vi "ABR3-Restore Defaults.vi"(7 "User":string) -> (4 "Params":T2={"CAP or ABR"=enum."ABR", "Stimulus"={"Ear"=enum."Left", "Waveform"=enum."TONE PIP", "Frequency (kHz)"="4", "Rep rate (/sec)"=30.0, "Alternate Polarity"=TRUE, "WavFiles"="", "Level (dB SPL)"=30.0, "WavFolder"=path "", "Chirp"={"Type"=enum."AN latency-corrected", "Duration (ms)"=0.0, "Fmin (kHz)"=0.0, "Fmax (kHz)"=0.0, "precompensate"=FALSE}, "Noise"={"Seed"=0, "InvFilt"=FALSE, "AWeight"=FALSE, "afile"=path "", "Filter"={"Type"=enum."Lowpass", "CF (kHz)"=0.0, "BW (kHz)"=0.0, "Cascade"=FALSE, "Quadrature"=FALSE, "Scale Factor"=0.0, "Stages"=[], "Class"=enum."Elliptic", "Order"=0, "BWUnits"=enum."Linear"}}}, "Masker"={"Filter"={"Type"=enum."Lowpass", "CF (kHz)"=0.0, "BW (kHz)"=0.0, "Cascade"=FALSE, "Quadrature"=FALSE, "Scale Factor"=0.0, "Stages"=[], "Class"=enum."Elliptic", "Order"=0, "BWUnits"=enum."Linear"}, "Use masker"=FALSE, "Level"={"Level"=0.0, "Units"=enum."dB atten", "Max"=0.0, "Multiplier"=0.0, "Cal File"=path "", "Cal"={"Freq (Hz)"=[], "Mag (dB SPL)"=[], "Phase (deg)"=[]}}, "Audiogram Comp"=FALSE, "Audiogram File"=path "", "InvFilt"=FALSE}, "Sequence"={"Start (dB)"=20, "Stop (dB)"=80, "Step (dB)"=5, "Var"=enum."Signal", "Order"=enum."Sequential"}, "Controls"={"on"=FALSE, "value"=0.0, "spacing"=0}, "Response"={"Gain"=10000, "Averages"=512, "Window (ms)"=8.5, "Thr Fast Steps"=1.5, "AI Fs"=25000.0}, "Hidden"={"AO Samp Rate Hz"=100000.0, "Duration (ms)"=5.0, "Ramp (ms)"=0.5, "Click width (us)"=100.0}} {"Response"."Thr Fast Steps" format="%.2f"; "Response"."Window (ms)" format="%.2f"; "Sequence"."Start (dB)" step=5}, 6 "Threshold Estimation":T1, 8 "settings":path=path "C:/Users/engr/Documents/EPL/CFTS/ABR/test.ini")   [LabVIEW 2020]
uses:
  TypeDefs/ABR3-Parameters.ctl
  TypeDefs/ABR3-Stimulus.ctl
  epl-vi-lib/Utility VIs/Type Defs/Left-Right ring.ctl
  TypeDefs/ABR-Waveform Enum.ctl
  epl-vi-lib/Signal Synthesis VIs/Controls/Advanced Filter XCtl/Advanced Filter XCtl.xctl
  TypeDefs/ABR3-Masker Spec.ctl
  epl-vi-lib/Signal Synthesis VIs/Controls/Level XCtl/Level XCtl.xctl
  TypeDefs/ABR3-Sequence Spec.ctl
  TypeDefs/ABR3-Controls.ctl
  TypeDefs/ABR3-Response.ctl
  TypeDefs/ABR3-Hidden Params.ctl
  Threshold Estimation VIs/ABR3-Threshold Estimation Parameters.ctl
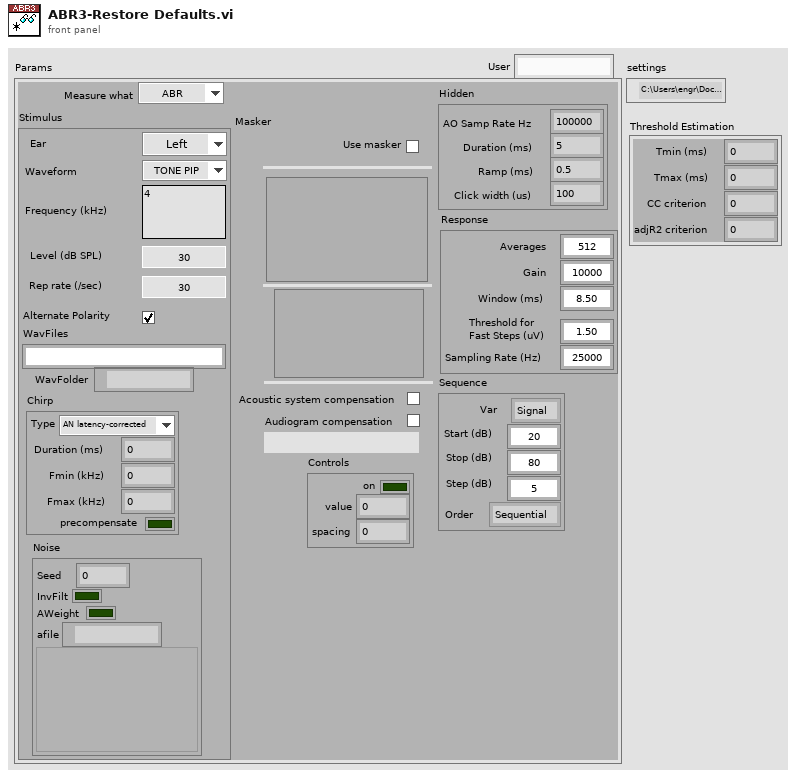
[diagram p1: front panel]
types:
  T1 = typedef "ABR3-Threshold Estimation Parameters.ctl" = cluster{"Tmin (ms)":dbl, "Tmax (ms)":dbl, "CC criterion":dbl, "adjR2 criterion":dbl}
  T2 = typedef "ABR3-Parameters.ctl" = cluster{"CAP or ABR":enum16{"CAP", "ABR"}, "Stimulus":T3, "Masker":T7, "Sequence":T9, "Controls":T10, "Response":T11, "Hidden":T12}
  T3 = typedef "ABR3-Stimulus.ctl" = cluster{"Ear":T4, "Waveform":T5, "Frequency (kHz)":string, "Rep rate (/sec)":dbl, "Alternate Polarity":bool, "WavFiles":string, "Level (dB SPL)":dbl, "WavFolder":path, "Chirp":cluster{"Type":enum16{"AN latency-corrected", "Arbitrary"}, "Duration (ms)":dbl, "Fmin (kHz)":dbl, "Fmax (kHz)":dbl, "precompensate":bool}, "Noise":cluster{"Seed":i32, "InvFilt":bool, "AWeight":bool, "afile":path, "Filter":cluster{"Type":enum16{"Lowpass", "Highpass", "Bandpass", "Bandstop", "OFF"}, "CF (kHz)":dbl, "BW (kHz)":dbl, "Cascade":bool, "Quadrature":bool, "Scale Factor":dbl, "Stages":cluster{"IIR Filter":cluster{"filter structure":enum32{"IIR 2nd Order", "IIR 4th Order"}, "Reverse Coefficients":dbl[], "Forward Coefficients":dbl[]}, "State":dbl[]}[], "Class":enum16{"Elliptic", "Butterworth"}, "Order":i32, "BWUnits":T6}}}
  T4 = typedef "Left-Right ring.ctl" = enum16{"Right", "Left"}
  T5 = typedef "ABR-Waveform Enum.ctl" = enum16{"TONE PIP", "CLICK", "FILE", "CHIRP", "NOISE", "VERHULST"}
  T6 = typedef "Filter-Bandwidth Units.ctl" = enum16{"Linear", "Octaves", "Min-Max"}
  T7 = typedef "ABR3-Masker Spec.ctl" = cluster{"Filter":cluster{"Type":enum16{"Lowpass", "Highpass", "Bandpass", "Bandstop", "OFF"}, "CF (kHz)":dbl, "BW (kHz)":dbl, "Cascade":bool, "Quadrature":bool, "Scale Factor":dbl, "Stages":cluster{"IIR Filter":cluster{"filter structure":enum32{"IIR 2nd Order", "IIR 4th Order"}, "Reverse Coefficients":dbl[], "Forward Coefficients":dbl[]}, "State":dbl[]}[], "Class":enum16{"Elliptic", "Butterworth"}, "Order":i32, "BWUnits":T6}, "Use masker":bool, "Level":cluster{"Level":dbl, "Units":T8, "Max":dbl, "Multiplier":dbl, "Cal File":path, "Cal":cluster{"Freq (Hz)":dbl[], "Mag (dB SPL)":dbl[], "Phase (deg)":dbl[]}}, "Audiogram Comp":bool, "Audiogram File":path, "InvFilt":bool}
  T8 = typedef "Level Units.ctl" = enum16{"dB atten", "dB SPL", "dB re 1 Vrms", "dB V/Hz½", "mW", "dB HL", "Volts", "dB mW"}
  T9 = typedef "ABR3-Sequence Spec.ctl" = cluster{"Start (dB)":i32, "Stop (dB)":i32, "Step (dB)":i32, "Var":enum16{"Signal", "Masker"}, "Order":enum16{"Sequential", "Random"}}
  T10 = typedef "ABR3-Controls.ctl" = cluster{"on":bool, "value":dbl, "spacing":i32}
  T11 = typedef "ABR3-Response.ctl" = cluster{"Gain":i32, "Averages":i32, "Window (ms)":sgl, "Thr Fast Steps":sgl, "AI Fs":dbl}
  T12 = typedef "ABR3-Hidden Params.ctl" = cluster{"AO Samp Rate Hz":dbl, "Duration (ms)":dbl, "Ramp (ms)":dbl, "Click width (us)":dbl}
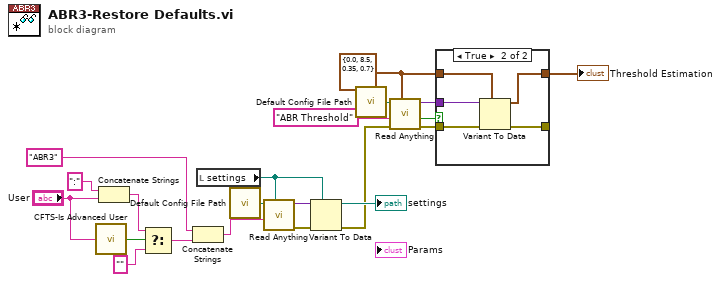
[diagram p0: block diagram]
diagram:
  w3 = T1 {"Tmin (ms)"=0.0, "Tmax (ms)"=8.5, "CC criterion"=0.35, "adjR2 criterion"=0.7} ("Threshold Estimation")
  n1 = call "CFTS-Is Advanced User.vi"("Experimenter"="User") -> ("Advanced user"=w17:bool)
  n2 = Concatenate Strings(":" ("string"), "User") -> (w14:string)
  n3 = Select(t=w14, s=w17, f="") -> (s? t:f=w12:string)
  n4 = Concatenate Strings("ABR3" ("Section Name (Name of \"Type of Anything\")"), w12) -> (w10:string)
  n5 = local read "settings"() -> (w19:path)
  n6 = call "Default Config File Path.vi"() -> ("Default config file name"=w20:path)
  n7 = call "Read Anything.vi"("Type of Anything"=w19, "Section Name (Name of \"Type of Anything\")"=w10, "Path (dialog)"=w20) -> ("Error Out"=w9:errorcluster, "Anything"=w21:variant)  [unwired: 6 in, 1 out]
  n8 = Variant To Data(error in=w9, type=w19, Variant=w21) -> (data=→"settings":path, error out=w2:errorcluster)
  n9 = call "Default Config File Path.vi"() -> ("Default config file name"=w8:path)
  n10 = call "Read Anything.vi"("Type of Anything"=w3, "Error In"=w2, "Section Name (Name of \"Type of Anything\")"="ABR Threshold" ("Section Name (Name of \"Type of Anything\")"), "Path (dialog)"=w8) -> ("Error Out"=w4:errorcluster, "Found?"=w6:bool, "Anything"=w5:variant)  [unwired: 5 in]
  n11 = case shown="True" w6 {
    tunnel: w5 -> [_ w27]
    tunnel: w3 -> [w23 w26]
    tunnel: w4 -> [w22 w28]
    tunnel: [w23 w25] -> w1
    tunnel: [w22 w24] -> _
    frame False {
    }
    frame True {
      n12 = Variant To Data(error in=w28, type=w26, Variant=w27) -> (data=w25:T1, error out=w24:errorcluster)
    }
  }
  "Threshold Estimation" <- w1
